vi "Climb Loop.vi"(0 "ClimbMotor":T12={"DeviceStatus"={"status"=FALSE, "code"=0, "source"=""}, "Type"=enum."PWM", "PWM"={"Digital Module"=enum."Digital Module 1", "PWM Channel"=enum."Invalid", "DeadBand"={"Name"="", "maxPositivePwm"=0, "minPositivePwm"=0, "centerPwm"=0, "maxNegativePwm"=0, "minNegativePwm"=0, "angularRange"=0}}, "CAN"={"Device Number"=0, "Control Mode"=enum."Percent VBus", "Semaphore"=refnum, "Max Vout"=12.0}, "Invert"=FALSE, "TransformRef"=refnum, "InvTransformRef"=refnum}, 1 "SkyHome":T7, 2 "Slapper":T9={"DevStatus"={"status"=FALSE, "code"=0, "source"=""}, "Solenoid Module"=enum."Solenoid Module 1", "Forward Solenoid Channel"=enum."Invalid", "Reverse Solenoid Channel"=enum."Invalid"}, 3 "Climb Step In":T1, 4 "Climb Step In2":T1, 5 "Time In":dbl, 6 "ClimbEncoder":T19={"DevStatus"={"status"=FALSE, "code"=0, "source"=""}, "EncoderIndex"=enum."Invalid", "CounterIndex"=enum."Invalid", "DistancePerCount"=1.0, "Decoding Type"=enum."4x"}, 7 "Rung counter in":i32, 8 "BrakeServo":T3={"DeviceStatus"={"status"=FALSE, "code"=0, "source"=""}, "Digital Module"=enum."Digital Module 1", "PWM Channel"=enum."Invalid", "DeadBand"={"Name"="", "maxPositivePwm"=0, "minPositivePwm"=0, "centerPwm"=0, "maxNegativePwm"=0, "minNegativePwm"=0, "angularRange"=0}}, 10 "PullUp":T9={"DevStatus"={"status"=FALSE, "code"=0, "source"=""}, "Solenoid Module"=enum."Solenoid Module 1", "Forward Solenoid Channel"=enum."Invalid", "Reverse Solenoid Channel"=enum."Invalid"}, 11 "array":i32[](array[numeric]), 12 "ClimbCurrent":T16, 13 "rt fifo":refnum<k33>, 15 "Auto Ascent Log Enable":bool=TRUE, 17 "time ref":dbl, 18 "Climb mode In":enum16{"Wait", "Automatic", "Manual", "Abort"}(ring)) -> (9 "Rung counter out":i32, 14 "Climb Step Out":T1, 16 "# elements":u32, 19 "Time Out":dbl)   [LabVIEW 2012]
uses:
  <vilib>/Rock Robotics/WPI/Encoder/WPI_EncoderDevRef.ctl
  <vilib>/Rock Robotics/SystemInterfaces/Encoder/FPGA_EncoderIdx.ctl
  <vilib>/Rock Robotics/SystemInterfaces/Counter/FPGA_CounterCtrSystemIndex.ctl
  <vilib>/Rock Robotics/WPI/Encoder/WPI_EncoderType.ctl
  <vilib>/Rock Robotics/WPI/AnalogChannel/WPI_AnalogChannelDevRef.ctl
  <vilib>/Rock Robotics/SystemInterfaces/Typedef/FPGA_TypedefAnalogModule.ctl
  <vilib>/Rock Robotics/SystemInterfaces/AI/FPGA_AIChannel.ctl
  <vilib>/Rock Robotics/WPI/Solenoid/WPI_SolenoidDevRef.ctl
  <vilib>/Rock Robotics/SystemInterfaces/Typedef/FPGA_TypedefSolenoidModule.ctl
  <vilib>/Rock Robotics/WPI/Solenoid/WPI_SolenoidChannel.ctl
  <vilib>/Rock Robotics/WPI/MotorControl/WPI_MotorControlDeviceRef.ctl
  <vilib>/Rock Robotics/SystemInterfaces/Typedef/FPGA_TypedefDigitalModule.ctl
  <vilib>/Rock Robotics/SystemInterfaces/DIO/FPGA_DIOPWMChannel.ctl
  <vilib>/Rock Robotics/WPI/PWM/WPI_PWMDeadband.ctl
  <vilib>/Rock Robotics/WPI/CAN/Jaguar/SubVIs/WPI_CANJaguar_ControlMode.ctl
  <vilib>/Rock Robotics/WPI/PWM/WPI_PWMTransform_ConPane.ctl
  climb_step_state.ctl
  <vilib>/Rock Robotics/WPI/DigitalInput/WPI_DigitalInputDevRef.ctl
  <vilib>/Rock Robotics/SystemInterfaces/DIO/FPGA_DIOChannel.ctl
  <vilib>/Rock Robotics/WPI/PWM/Servo/WPI_ServoDeviceRef.ctl
  <vilib>/Rock Robotics/WPI/Solenoid/WPI_SolenoidValue.ctl
  <vilib>/Rock Robotics/WPI/Solenoid/WPI_SolenoidSetEnum.vi
panel:
  out "Prev":T1
  in  "s":bool
  out "Current":dbl(graph)
  in  "Tab Control":T2(tab)
  in  "Auto Flip Speed":dbl=-0.2
  in  "distance to flip":dbl=-630.0
  in  "Man Flip Speed":dbl=-0.75
  out "Distance Flip":dbl
  in  "Target extend dist":dbl=1000.0
  in  "Motor Coerce":dbl=0.85
  out "At Lo":bool
  out "At Hi":bool
  in  "Near Limit":dbl=400.0
  in  "Speed near Lim Up":dbl=0.2
  in  "Precision":bool=TRUE
  out "Distance":dbl
  in  "Speed near Lim Dn":dbl=0.11
  out "state":bool
  in  "reset":bool
  in  "wait":dbl=2.0
  in  "Target extend dist 2":dbl=2735.0
  out "state 2":bool
  out "At Hi 2":bool
  out "At Lo 2":bool
  in  "Speed near Lim Dn 2":dbl=0.11
  out "Distance 2":dbl
  in  "Speed near Lim Up 2":dbl=0.2
  in  "Near Limit 2":dbl=400.0
  in  "Motor Coerce 2":dbl=0.85
  in  "Retract Test Dist":dbl=2450.0
  in  "delay post slap":dbl=2.0
  out "Auto Current":dbl(graph)
  in  "Current sensor load 2":dbl=0.5
  out "Voltage":dbl
  in  "Distance desired to\nretract tail hook completely 2":dbl=-650.0
  out "Distance Retracted":dbl
  out "Dist Used":dbl
  in  "L3 offset":dbl=20.0
  out "State":enum16{"Engaged", "Untension", "Disengaged"}(ring)
  in  "Brake Delay":dbl=0.2
  in  "Servo Disengage":i32
  in  "Untension Speed":dbl=-0.1
  in  "Reverse Time":dbl=0.4
  in  "Servo Engage":i32=120
  in  "Slow Retract":dbl=-0.25
  in  "Slow Extend":dbl=0.25
  in  "Climb Extend Speed":dbl=1.0
  in  "Climb Retract Speed":dbl=-0.9
  out "State 2":enum16{"Engaged", "Untension", "Disengaged"}(ring)
  in  "Servo Disengage 2":i32
  in  "Servo Engage 2":i32=120
  in  "Brake Delay 2":dbl=0.2
  in  "Reverse Time 2":dbl=0.4
  in  "Untension Speed 2":dbl=-0.1
  out "SkyHook is Home":bool
  out "Sky Enc":dbl
  out "Climb Started?":bool
  # "Encoder Displacement\n110 counts ~ 1 inch\n7 counts ~ 1/16 inch\n40 counts ~ Tooth-tooth on brake wheel"
  # "was -0.18 at Champs"
  # "It is a delay to allow the robot to stop \nswinging after a T-Rex pull-up, prior to \nextending the ShyHook to max distance.\n\nThis delay only affects level 2, not level 3."
  # "Distance desired to \nretract (enough to detect if\nwe have weight on current sensor\nin next case) 2"
  # "BRAKE"
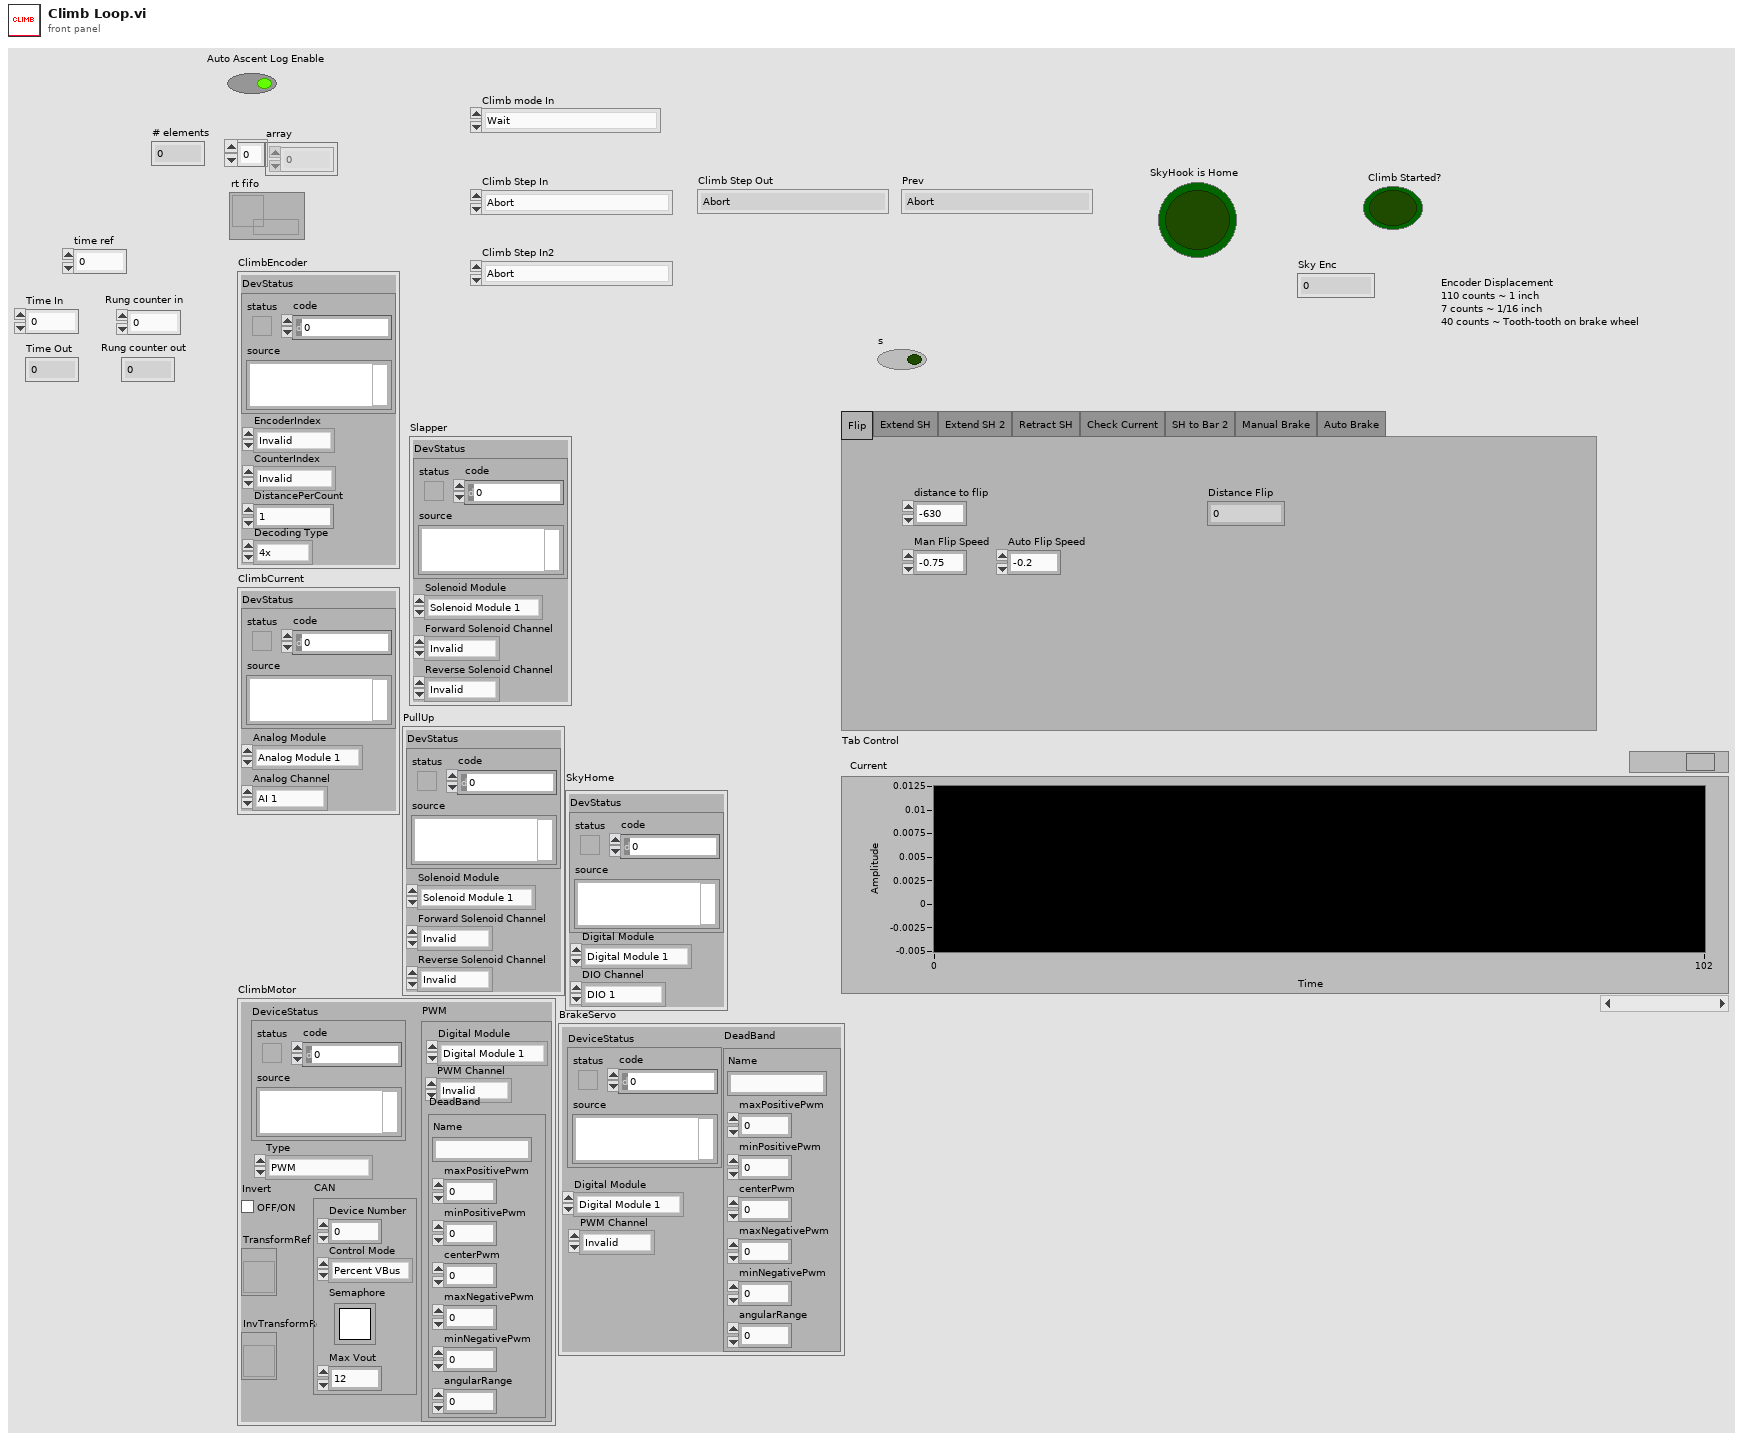
[diagram p1: front panel]
types:
  T1 = typedef "climb_step_state.ctl" = enum16{"Abort", "Approach Bar", "Approach +", "Climb Step 1", "Climb Step 2", "Climb Step 3", "Climb Step 4", "Climb Step 5", "Climb Step 6", "Climb Step 7", "Check Finished", "Check Continue"}
  T2 = enum32{"Flip", "Extend SH", "Extend SH 2", "Retract SH", "Check Current", "SH to Bar 2", "Manual Brake", "Auto Brake"}
  T3 = typedef "WPI_ServoDeviceRef.ctl" = cluster{"DeviceStatus":errorcluster, "Digital Module":T4, "PWM Channel":T5, "DeadBand":T6}
  T4 = typedef "FPGA_TypedefDigitalModule.ctl" = enum16{"Digital Module 1", "Digital Module 2"}
  T5 = typedef "FPGA_DIOPWMChannel.ctl" = enum8{"PWM 1", "PWM 2", "PWM 3", "PWM 4", "PWM 5", "PWM 6", "PWM 7", "PWM 8", "PWM 9", "PWM 10", "Invalid"}
  T6 = typedef "WPI_PWMDeadband.ctl" = cluster{"Name":string, "maxPositivePwm":i32, "minPositivePwm":i32, "centerPwm":i32, "maxNegativePwm":i32, "minNegativePwm":i32, "angularRange":u16}
  T7 = typedef "WPI_DigitalInputDevRef.ctl" = cluster{"DevStatus":errorcluster, "DIO Channel":T8, "Digital Module":T4}
  T8 = typedef "FPGA_DIOChannel.ctl" = enum8{"DIO 1", "DIO 2", "DIO 3", "DIO 4", "DIO 5", "DIO 6", "DIO 7", "DIO 8", "DIO 9", "DIO 10", "DIO 11", "DIO 12", "DIO 13", "DIO 14", "Invalid"}
  T9 = typedef "WPI_SolenoidDevRef.ctl" = cluster{"DevStatus":errorcluster, "Solenoid Module":T10, "Forward Solenoid Channel":T11, "Reverse Solenoid Channel":T11}
  T10 = typedef "FPGA_TypedefSolenoidModule.ctl" = enum16{"Solenoid Module 1", "Solenoid Module 2"}
  T11 = typedef "WPI_SolenoidChannel.ctl" = enum8{"Solenoid 1", "Solenoid 2", "Solenoid 3", "Solenoid 4", "Solenoid 5", "Solenoid 6", "Solenoid 7", "Solenoid 8", "Invalid"}
  T12 = typedef "WPI_MotorControlDeviceRef.ctl" = cluster{"DeviceStatus":errorcluster, "Type":enum16{"PWM", "CAN"}, "PWM":cluster{"Digital Module":T4, "PWM Channel":T5, "DeadBand":T6}, "CAN":cluster{"Device Number":u8, "Control Mode":T13, "Semaphore":T14, "Max Vout":dbl}, "Invert":bool, "TransformRef":T15, "InvTransformRef":T15}
  T13 = typedef "WPI_CANJaguar_ControlMode.ctl" = enum8{"Percent VBus", "Current", "Speed", "Position", "Voltage"}
  T14 = typedef "Semaphore RefNum" = refnum<k1>
  T15 = typedef "WPI_PWMTransform_ConPane.ctl" = refnum<vi>
  T16 = typedef "WPI_AnalogChannelDevRef.ctl" = cluster{"DevStatus":errorcluster, "Analog Module":T17, "Analog Channel":T18}
  T17 = typedef "FPGA_TypedefAnalogModule.ctl" = enum16{"Analog Module 1", "Analog Module 2"}
  T18 = typedef "FPGA_AIChannel.ctl" = enum8{"AI 1", "AI 2", "AI 3", "AI 4", "AI 5", "AI 6", "AI 7", "AI 8", "Invalid"}
  T19 = typedef "WPI_EncoderDevRef.ctl" = cluster{"DevStatus":errorcluster, "EncoderIndex":T20, "CounterIndex":T21, "DistancePerCount":dbl, "Decoding Type":T22}
  T20 = typedef "FPGA_EncoderIdx.ctl" = enum8{"Enc 0", "Enc 1", "Enc 2", "Enc 3", "Invalid"}
  T21 = typedef "FPGA_CounterCtrSystemIndex.ctl" = enum8{"Ctr 0", "Ctr 1", "Ctr 2", "Ctr 3", "Ctr 4", "Ctr 5", "Ctr 6", "Ctr 7", "Invalid"}
  T22 = typedef "WPI_EncoderType.ctl" = enum16{"1x", "2x", "4x"}
  T23 = typedef "WPI_SolenoidValue.ctl" = enum16{"Off", "On", "Forward", "Reverse"}
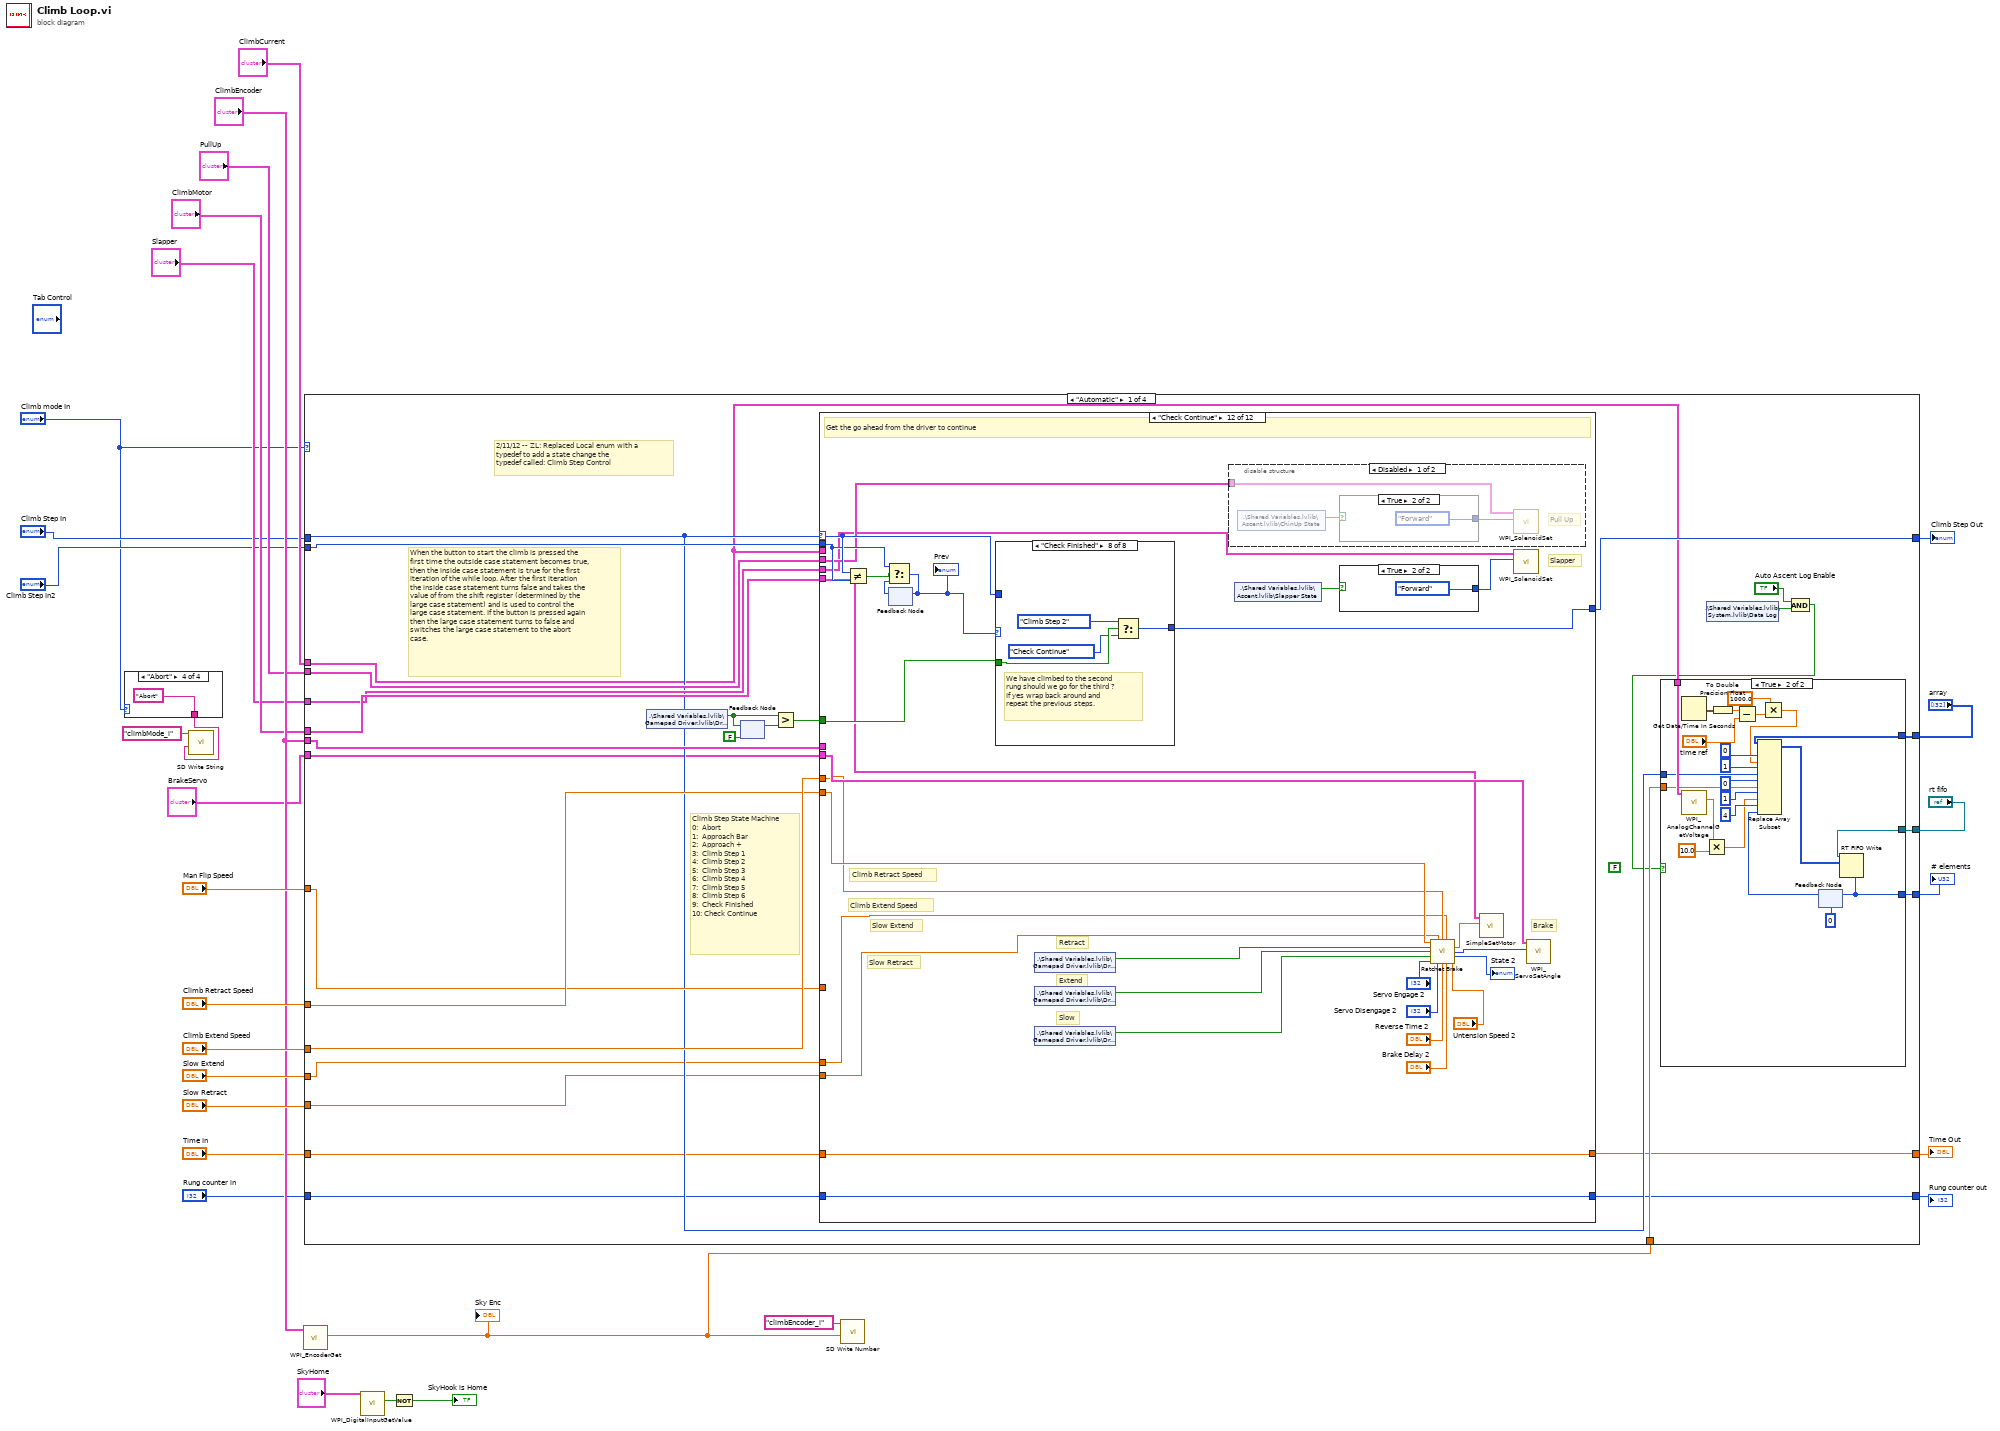
[diagram p0: block diagram]
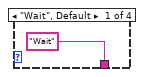
[diagram p2: hidden frame]
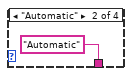
[diagram p3: hidden frame]
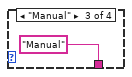
[diagram p4: hidden frame]
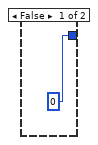
[diagram p5: hidden frame]
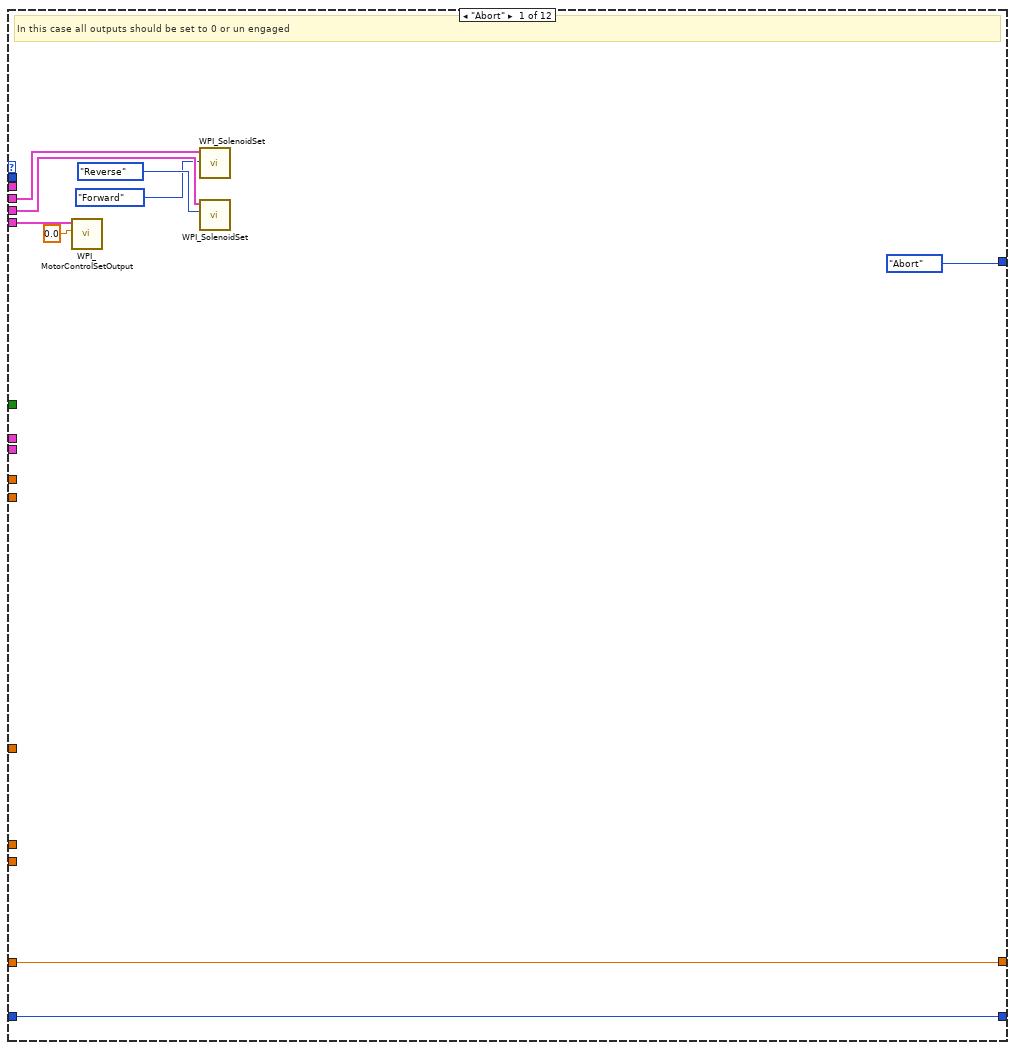
[diagram p6: hidden frame]
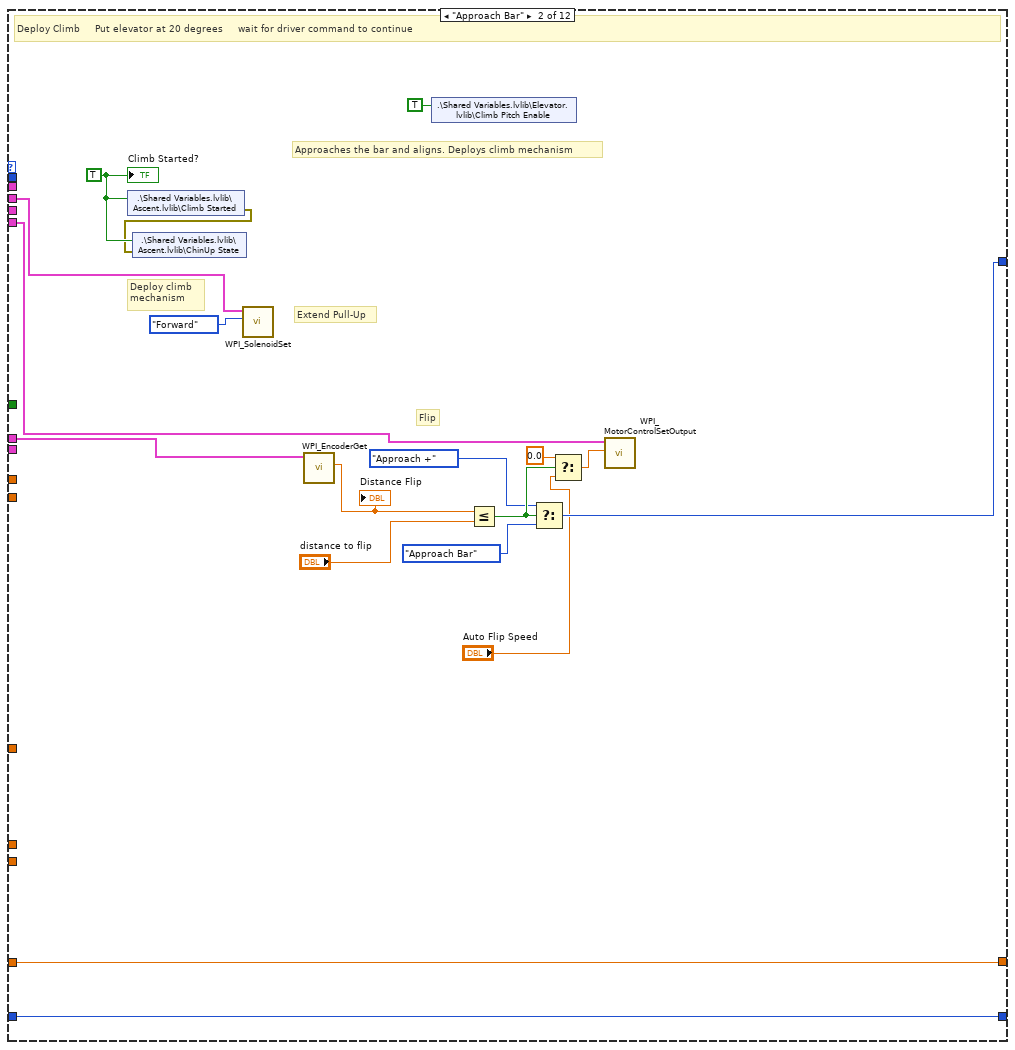
[diagram p7: hidden frame]
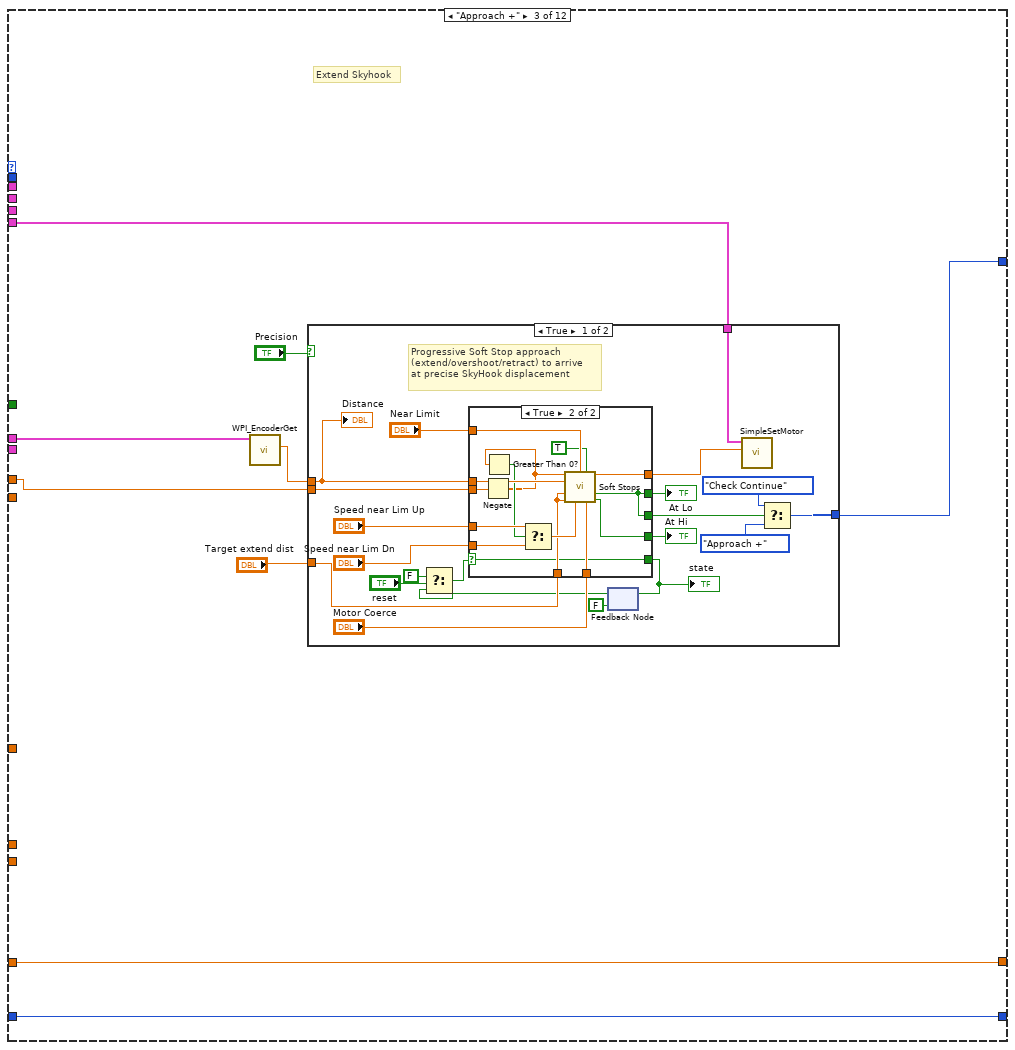
[diagram p8: hidden frame]
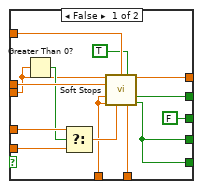
[diagram p9: hidden frame]
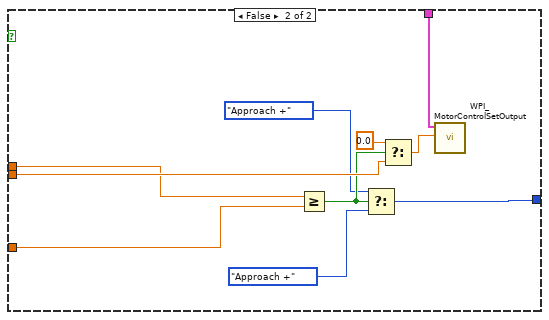
[diagram p10: hidden frame]
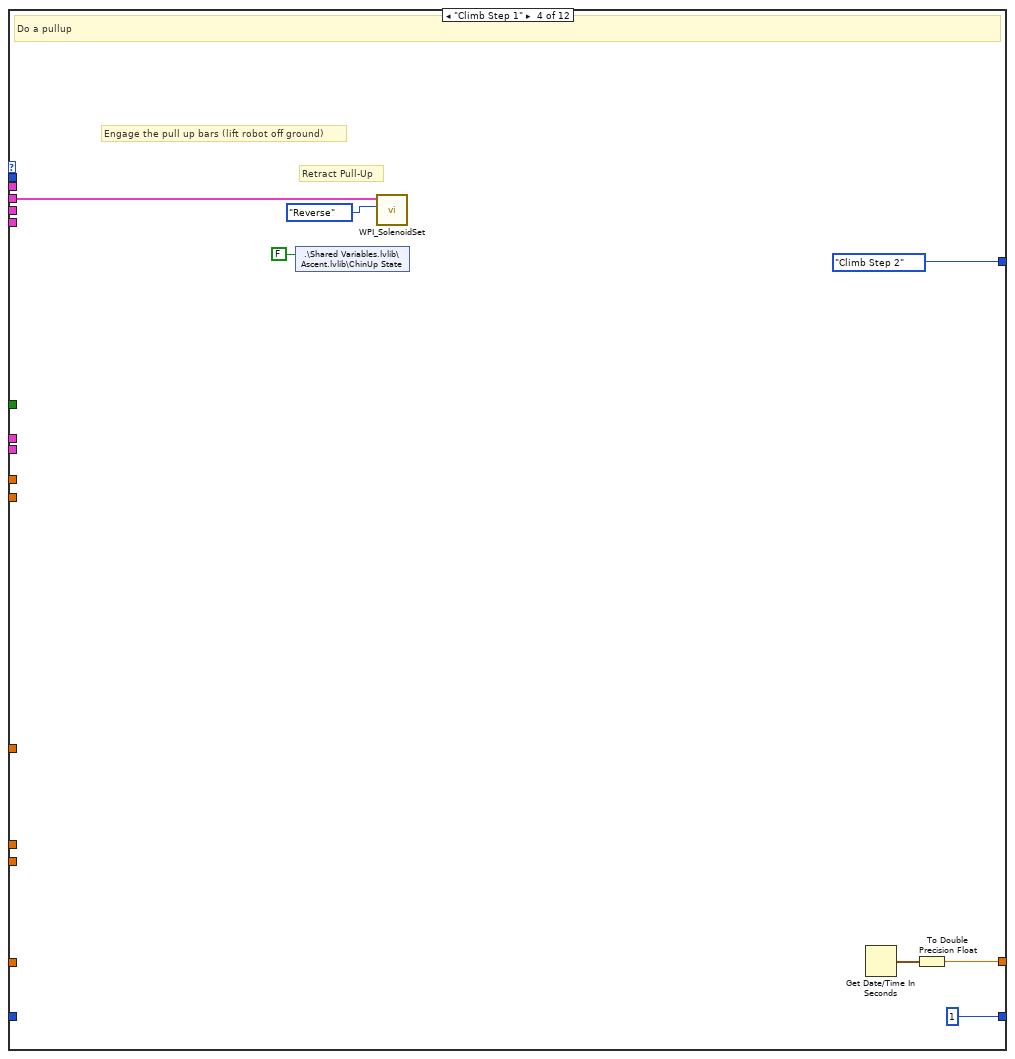
[diagram p11: hidden frame]
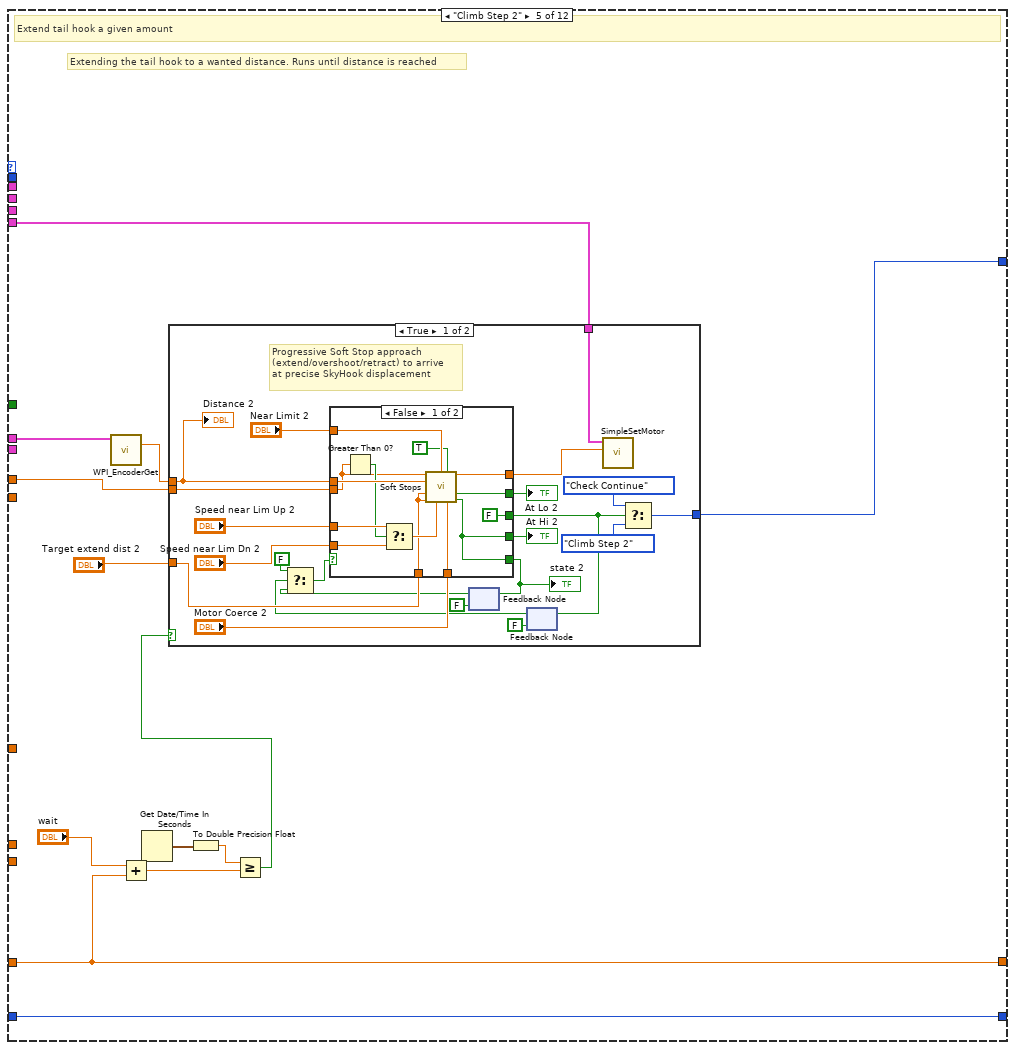
[diagram p12: hidden frame]
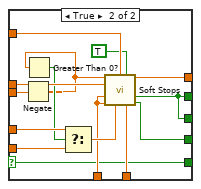
[diagram p13: hidden frame]
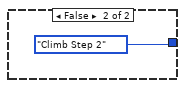
[diagram p14: hidden frame]
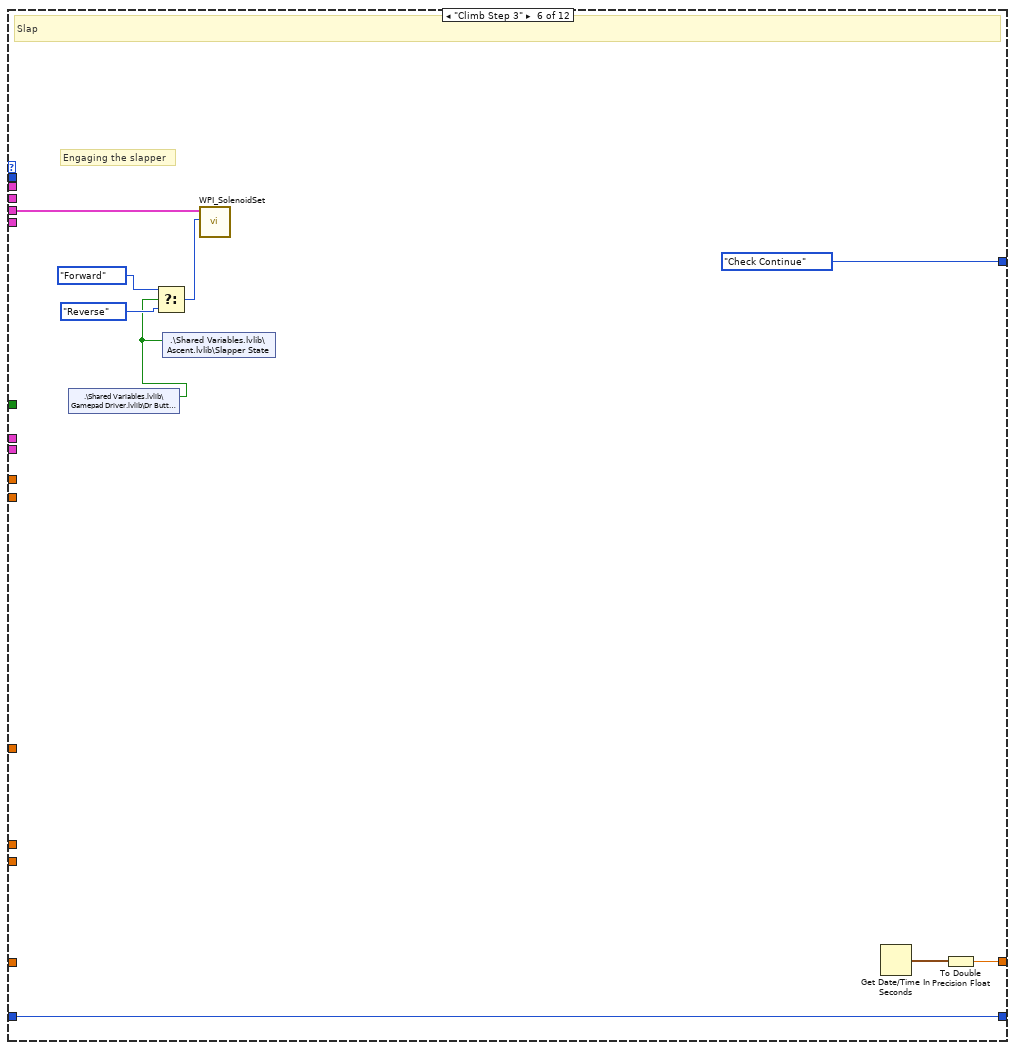
[diagram p15: hidden frame]
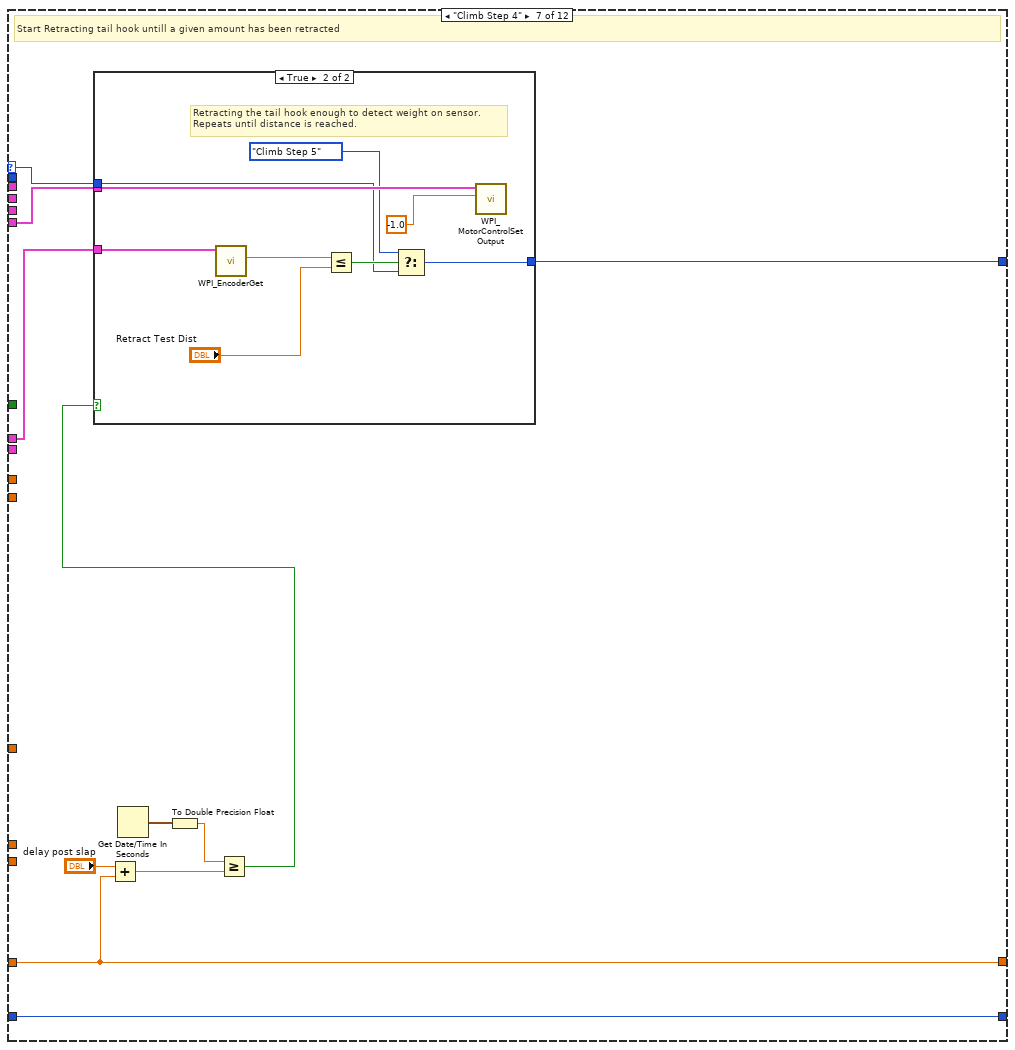
[diagram p16: hidden frame]
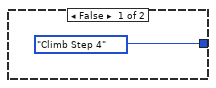
[diagram p17: hidden frame]
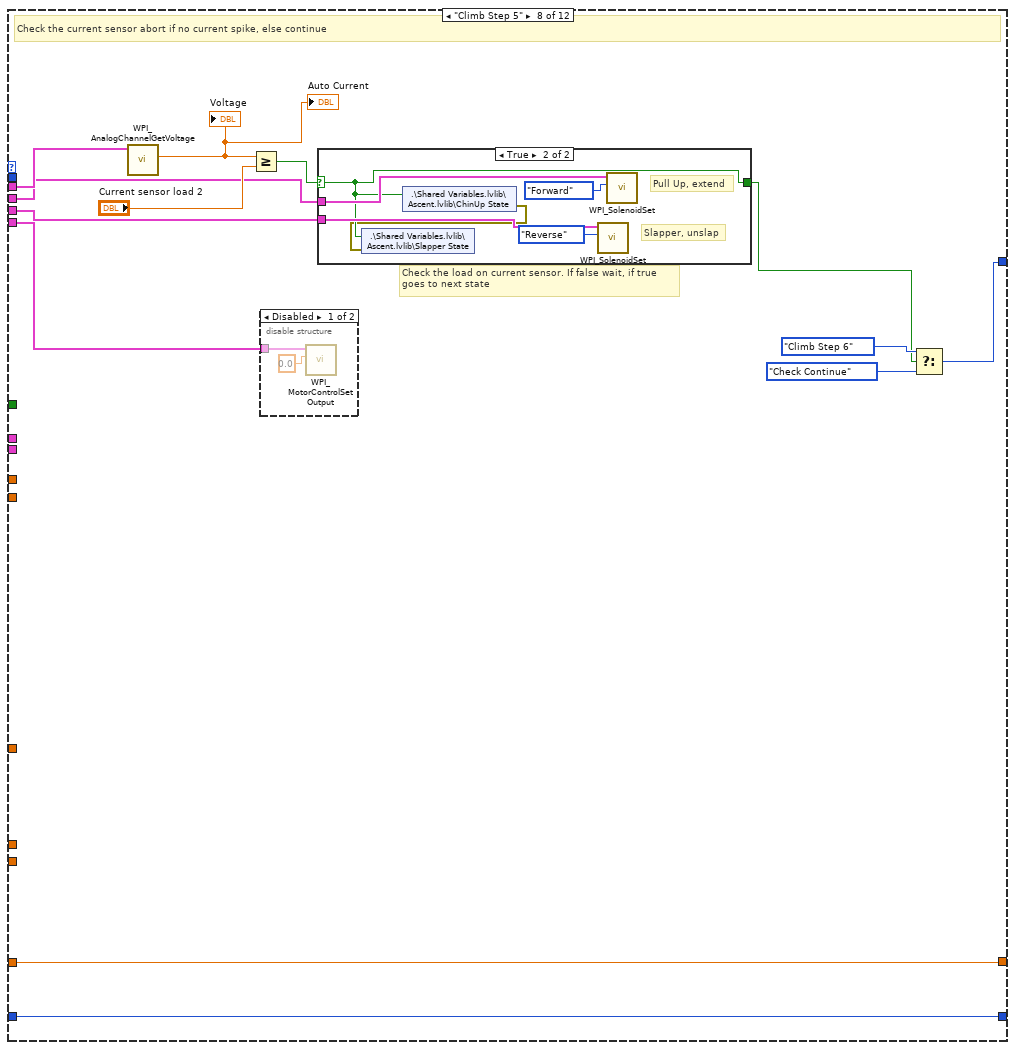
[diagram p18: hidden frame]
diagram:
  n1 = case shown="\"Abort\"" "Climb mode In" {
    tunnel: ["Wait" "Automatic" "Manual" "Abort"] -> w28
    frame "Wait", Default {
    }
    frame "Automatic" {
    }
    frame "Manual" {
    }
    frame "Abort" {
    }
  }
  n2 = call <vilib>:"SD Write String.vi"("String"=w28, "Name"="climbMode_i") -> ()  [unwired: 8 in, 2 out]
  n3 = call <vilib>:"WPI_EncoderGet.vi"("EncoderDevRef"="ClimbEncoder") -> ("Distance"=w1:dbl)  [unwired: 5 in, 5 out]
  "Sky Enc" <- w1
  n4 = case shown="\"Automatic\"" "Climb mode In" {
    tunnel: "PullUp" -> [w62 _ _ w438]
    tunnel: "ClimbMotor" -> [w61 _ _ w437]
    tunnel: "ClimbEncoder" -> [w60 _ _ _]
    tunnel: "Slapper" -> [w59 _ w421 w439]
    tunnel: "ClimbCurrent" -> [w43 _ _ w428]
    tunnel: [w58 climb_step_state."Abort" ("Climb Step") climb_step_state."Approach Bar" ("Climb Step") climb_step_state."Abort" ("Climb Step")] -> w13
    tunnel: "Climb Step In" -> [w45 _ _ _]
    tunnel: "Climb Step In2" -> [w57 _ _ _]
    tunnel: "Climb Extend Speed" -> [w56 _ _ w435]
    tunnel: "Climb Retract Speed" -> [w55 _ _ w434]
    tunnel: "Man Flip Speed" -> [w54 _ _ w433]
    tunnel: "Slow Extend" -> [w40 _ _ w432]
    tunnel: "Slow Retract" -> [w39 _ _ w431]
    tunnel: "BrakeServo" -> [w41 _ w420 w429]
    tunnel: "array" -> [w49 _ _ _]
    tunnel: [w48 u32 0 ("# elements") u32 0 ("# elements") u32 0 ("# elements")] -> w7
    tunnel: w1 -> [w44 _ _ _]
    tunnel: "rt fifo" -> [w42 _ _ _]
    tunnel: [w38 w413 w417 w425] -> w5
    tunnel: "Time In" -> [w37 w413 w417 w425]
    tunnel: [w36 w414 w418 w426] -> w3
    tunnel: "Rung counter in" -> [w35 w414 w418 w426]
    frame "Automatic" {
      (unwired) FALSE
      # "Climb Step State Machine\n0:  Abort\n1:  Approach Bar\n2:  Approach +\n3:  Climb Step 1\n4:  Climb Step 2\n5:  Climb Step 3\n6:  Climb Step 4\n7:  Climb Step 5\n8:  Climb Step 6\n9:  Check Finished\n10: Check Continue"
      # "2/11/12 -- ZL: Replaced Local enum with a \ntypedef to add a state change the \ntypedef called: Climb Step Control"
      # "When the button to start the climb is pressed the\nfirst time the outside case statement becomes true,\nthen the inside case statement is true for the first\niteration of the while loop. After the first iteration\nthe inside case statement turns false and takes the\nvalue of from the shift register (determined by the\nlarge case statement) and is used to control the \nlarge case statement. If the button is pressed again \nthen the large case statement turns to false and \nswitches the large case statement to the abort\ncase."
      n5 = shared-variable ".\\Shared Variables.lvlib\\Gamepad Driver.lvlib\\Dr Button 1"() -> (w53:bool)  [unwired: 1 in, 1 out]
      n6 = feedback-in #1(w53) -> ()
      n7 = feedback #1(FALSE ("Boolean")) -> (w52:bool)
      n8 = Greater?(x=w53, y=w52) -> (0:w51:bool)
      n9 = case shown="\"Check Continue\"" w45 {
        selector: w45 -> [_ _ _ _ _ _ w272 _ w319 _ _ w376]
        tunnel: w62 -> [w91 w113 _ w189 _ _ _ w293 w322 w336 _ w349]
        tunnel: [climb_step_state."Abort" ("Climb Step") w102 w116 climb_step_state."Climb Step 2" ("Climb Step") w190 climb_step_state."Check Continue" ("Climb Step") w273 w292 w320 w332 w342 w352] -> w58
        tunnel: w61 -> [w95 w111 w119 _ w193 _ w274 w286 w323 _ _ w357]
        tunnel: w60 -> [_ w110 w122 _ w192 _ w270 _ w326 _ _ _]
        tunnel: w59 -> [w93 _ _ _ _ w263 _ w294 _ _ _ w348]
        tunnel: w43 -> [_ _ _ _ _ _ _ w297 _ _ _ _]
        tunnel: w57 -> [_ _ _ _ _ _ _ _ _ _ _ w374]
        tunnel: w56 -> [_ _ w121 _ w191 _ _ _ _ _ _ w355]
        tunnel: w55 -> [_ _ _ _ _ _ _ _ _ _ _ w356]
        tunnel: w54 -> [_ _ _ _ _ _ _ _ _ _ _ _]
        tunnel: [w88 w99 w115 1 w202 w262 w271 w289 w315 w334 w340 w371] -> w36
        tunnel: w35 -> [w88 w99 w115 _ w202 w262 w271 w289 w315 w334 w341 w371]
        tunnel: [w87 w98 w114 w184 w197 w258 w269 w288 w318 w335 w339 w370] -> w38
        tunnel: w37 -> [w87 w98 w114 _ w197 _ w269 w288 w318 w335 w339 w370]
        tunnel: w51 -> [_ _ _ _ _ _ _ _ _ _ _ w369]
        tunnel: w41 -> [_ _ _ _ _ _ _ _ _ _ _ w358]
        tunnel: w40 -> [_ _ _ _ _ _ _ _ _ _ _ w354]
        tunnel: w39 -> [_ _ _ _ _ _ _ _ _ _ _ w353]
        frame "Abort" {
          # "In this case all outputs should be set to 0 or un engaged"
          n10 = call <vilib>:"WPI_MotorControlSetOutput.vi"("Output"=0.0, "MotorControlDevRef"=w95) -> ()  [unwired: 7 in, 3 out]
          n11 = call-poly <vilib>:"WPI_SolenoidSet.vi"("Value"=WPI_SolenoidValue."Forward", "SolenoidDevRef"=w91) -> ()  [unwired: 8 in, 2 out]
          n12 = call-poly <vilib>:"WPI_SolenoidSet.vi"("Value"=WPI_SolenoidValue."Reverse", "SolenoidDevRef"=w93) -> ()  [unwired: 8 in, 2 out]
        }
        frame "Approach Bar" {
          w97 = TRUE ("Climb Started?")
          # "Flip"
          # "Extend Pull-Up"
          # "Deploy climb \nmechanism"
          # "Approaches the bar and aligns. Deploys climb mechanism"
          # "Deploy Climb     Put elevator at 20 degrees     wait for driver command to continue"
          n13 = shared-variable ".\\Shared Variables.lvlib\\Ascent.lvlib\\Climb Started"(w97) -> (error out=w96:errorcluster)  [unwired: 1 in]
          n14 = shared-variable ".\\Shared Variables.lvlib\\Ascent.lvlib\\ChinUp State"(w97, error in=w96) -> ()  [unwired: 1 out]
          n15 = call-poly <vilib>:"WPI_SolenoidSet.vi"("Value"=WPI_SolenoidValue."Forward", "SolenoidDevRef"=w113) -> ()  [unwired: 8 in, 2 out]
          n16 = call <vilib>:"WPI_EncoderGet.vi"("EncoderDevRef"=w110) -> ("Distance"=w106:dbl)  [unwired: 5 in, 5 out]
          "Distance Flip" <- w106
          n17 = shared-variable ".\\Shared Variables.lvlib\\Elevator.lvlib\\Climb Pitch Enable"(TRUE ("Climb Pitch Enable")) -> ()  [unwired: 1 in, 1 out]
          n18 = Less Or Equal?(x=w106, y="distance to flip") -> (x <= y?=w105:bool)
          n19 = Select(t=climb_step_state."Approach +" ("Climb Step"), s=w105, f=climb_step_state."Approach Bar" ("Climb Step")) -> (s? t:f=w102:T1)
          n20 = Select(t=0.0, s=w105, f="Auto Flip Speed") -> (s? t:f=w107:dbl)
          n21 = call <vilib>:"WPI_MotorControlSetOutput.vi"("Output"=w107, "MotorControlDevRef"=w111) -> ()  [unwired: 7 in, 3 out]
          "Climb Started?" <- w97
        }
        frame "Approach +" {
          # "Extend Skyhook"
          n22 = call <vilib>:"WPI_EncoderGet.vi"("EncoderDevRef"=w122) -> ("Distance"=w120:dbl)  [unwired: 5 in, 5 out]
          n23 = case shown="True" "Precision" {
            tunnel: w121 -> [w131 w182]
            tunnel: w120 -> [w133 w181]
            tunnel: w119 -> [w140 w180]
            tunnel: "Target extend dist" -> [w132 w179]
            tunnel: [w141 w173] -> w116
            frame True {
              # "Progressive Soft Stop approach\n(extend/overshoot/retract) to arrive \nat precise SkyHook displacement"
              n24 = feedback #2(FALSE) -> (w124:bool)
              n25 = Select(t=FALSE, s="reset", f=w124) -> (s? t:f=w126:bool)
              n26 = case shown="True" w126 {
                selector: w126 -> [_ w162]
                tunnel: "Near Limit" -> [w157 w172]
                tunnel: "Motor Coerce" -> [w156 w171]
                tunnel: [FALSE ("At Hi") w160] -> w137
                tunnel: [w154 w169] -> w136
                tunnel: "Speed near Lim Up" -> [w152 w167]
                tunnel: "Speed near Lim Dn" -> [w151 w166]
                tunnel: w133 -> [w150 w165]
                tunnel: w132 -> [w148 w163]
                tunnel: w131 -> [w147 w159]
                tunnel: [w144 w162] -> w130
                tunnel: [w145 w160] -> w128
                tunnel: [w144 w161] -> w127
                frame False {
                  n27 = Greater Than 0?(x=w147) -> (x > 0?=w149:bool)
                  n28 = Select(t=w152, s=w149, f=w151) -> (s? t:f=w153:dbl)
                  n29 = call "Soft Stops.vi"("Motor In"=w147, "correlation"=TRUE, "Sense"=w150, "Lo Limit"=w148, "Hi Limit"=w148, "Speed near Limit"=w153, "Margin"=w157, "Motor Coerce"=w156) -> ("Motor Out"=w154:dbl, "At Lo"=w145:bool, "At Hi"=w144:bool)  [unwired: 5 in]
                }
                frame True {
                  n30 = Negate(x=w159) -> (-x=w158:dbl)
                  n31 = Greater Than 0?(x=w158) -> (x > 0?=w164:bool)
                  n32 = Select(t=w167, s=w164, f=w166) -> (s? t:f=w168:dbl)
                  n33 = call "Soft Stops.vi"("Motor In"=w158, "correlation"=TRUE, "Sense"=w165, "Lo Limit"=w163, "Hi Limit"=w163, "Speed near Limit"=w168, "Margin"=w172, "Motor Coerce"=w171) -> ("Motor Out"=w169:dbl, "At Lo"=w160:bool, "At Hi"=w161:bool)  [unwired: 5 in]
                }
              }
              "At Lo" <- w128
              "At Hi" <- w127
              "state" <- w130
              n34 = feedback-in #2(w130) -> ()
              n35 = call "SimpleSetMotor.vi"("Output"=w136, "MotorControlDevRef"=w140) -> ()  [unwired: 8 in, 2 out]
              n36 = Select(t=climb_step_state."Check Continue" ("Climb Step"), s=w137, f=climb_step_state."Approach +" ("Climb Step")) -> (s? t:f=w141:T1)
              "Distance" <- w133
            }
            frame False {
              n37 = Greater Or Equal?(x=w181, y=w179) -> (x >= y?=w176:bool)
              n38 = Select(t=climb_step_state."Approach +" ("Climb Step"), s=w176, f=climb_step_state."Approach +" ("Climb Step")) -> (s? t:f=w173:T1)
              n39 = Select(t=0.0, s=w176, f=w182) -> (s? t:f=w177:dbl)
              n40 = call <vilib>:"WPI_MotorControlSetOutput.vi"("Output"=w177, "MotorControlDevRef"=w180) -> ()  [unwired: 7 in, 3 out]
            }
          }
        }
        frame "Climb Step 1" {
          # "Retract Pull-Up"
          # "Engage the pull up bars (lift robot off ground)"
          # "Do a pullup"
          n41 = shared-variable ".\\Shared Variables.lvlib\\Ascent.lvlib\\ChinUp State"(FALSE ("ChinUp State")) -> ()  [unwired: 1 in, 1 out]
          n42 = call-poly <vilib>:"WPI_SolenoidSet.vi"("Value"=WPI_SolenoidValue."Reverse", "SolenoidDevRef"=w189) -> ()  [unwired: 8 in, 2 out]
          n43 = Get Date/Time In Seconds() -> (seconds since 1Jan1904=w185:timestamp)
          n44 = To Double Precision Float(number=w185) -> (double precision float=w184:dbl)
        }
        frame "Climb Step 2" {
          # "Extending the tail hook to a wanted distance. Runs until distance is reached"
          # "Extend tail hook a given amount"
          n45 = call <vilib>:"WPI_EncoderGet.vi"("EncoderDevRef"=w192) -> ("Distance"=w196:dbl)  [unwired: 5 in, 5 out]
          n46 = Add(x="wait", y=w197) -> (x+y=w199:dbl)
          n47 = Get Date/Time In Seconds() -> (seconds since 1Jan1904=w201:timestamp)
          n48 = To Double Precision Float(number=w201) -> (double precision float=w198:dbl)
          n49 = Greater Or Equal?(x=w198, y=w199) -> (x >= y?=w194:bool)
          n50 = case shown="True" w194 {
            tunnel: w191 -> [w213 _]
            tunnel: w196 -> [w215 _]
            tunnel: w193 -> [w221 _]
            tunnel: "Target extend dist 2" -> [w214 _]
            tunnel: [w222 climb_step_state."Climb Step 2" ("Climb Step")] -> w190
            frame True {
              # "Progressive Soft Stop approach\n(extend/overshoot/retract) to arrive \nat precise SkyHook displacement"
              n51 = feedback #3(FALSE) -> (w207:bool)
              n52 = feedback #4(FALSE) -> (w203:bool)
              n53 = Select(t=FALSE, s=w203, f=w207) -> (s? t:f=w208:bool)
              n54 = case shown="False" w208 {
                selector: w208 -> [_ w243]
                tunnel: "Near Limit 2" -> [w238 w253]
                tunnel: "Motor Coerce 2" -> [w237 w252]
                tunnel: [FALSE ("At Hi") w241] -> w204
                tunnel: [w235 w250] -> w218
                tunnel: "Speed near Lim Up 2" -> [w233 w248]
                tunnel: "Speed near Lim Dn 2" -> [w232 w247]
                tunnel: w215 -> [w231 w246]
                tunnel: w214 -> [w229 w244]
                tunnel: w213 -> [w228 w240]
                tunnel: [w225 w243] -> w212
                tunnel: [w226 w241] -> w210
                tunnel: [w225 w242] -> w209
                frame False {
                  n55 = Greater Than 0?(x=w228) -> (x > 0?=w230:bool)
                  n56 = Select(t=w233, s=w230, f=w232) -> (s? t:f=w234:dbl)
                  n57 = call "Soft Stops.vi"("Motor In"=w228, "correlation"=TRUE, "Sense"=w231, "Lo Limit"=w229, "Hi Limit"=w229, "Speed near Limit"=w234, "Margin"=w238, "Motor Coerce"=w237) -> ("Motor Out"=w235:dbl, "At Lo"=w226:bool, "At Hi"=w225:bool)  [unwired: 5 in]
                }
                frame True {
                  n58 = Negate(x=w240) -> (-x=w239:dbl)
                  n59 = Greater Than 0?(x=w239) -> (x > 0?=w245:bool)
                  n60 = Select(t=w248, s=w245, f=w247) -> (s? t:f=w249:dbl)
                  n61 = call "Soft Stops.vi"("Motor In"=w239, "correlation"=TRUE, "Sense"=w246, "Lo Limit"=w244, "Hi Limit"=w244, "Speed near Limit"=w249, "Margin"=w253, "Motor Coerce"=w252) -> ("Motor Out"=w250:dbl, "At Lo"=w241:bool, "At Hi"=w242:bool)  [unwired: 5 in]
                }
              }
              "At Lo 2" <- w210
              "At Hi 2" <- w209
              "state 2" <- w212
              n62 = feedback-in #3(w212) -> ()
              n63 = feedback-in #4(w204) -> ()
              n64 = call "SimpleSetMotor.vi"("Output"=w218, "MotorControlDevRef"=w221) -> ()  [unwired: 8 in, 2 out]
              n65 = Select(t=climb_step_state."Check Continue" ("Climb Step"), s=w204, f=climb_step_state."Climb Step 2" ("Climb Step")) -> (s? t:f=w222:T1)
              "Distance 2" <- w215
            }
            frame False {
            }
          }
        }
        frame "Climb Step 3" {
          # "Engaging the slapper"
          # "Slap"
          n66 = shared-variable ".\\Shared Variables.lvlib\\Gamepad Driver.lvlib\\Dr Button 12"() -> (w255:bool)  [unwired: 1 in, 1 out]
          n67 = Select(t=WPI_SolenoidValue."Forward" ("Value"), s=w255, f=WPI_SolenoidValue."Reverse" ("Value")) -> (s? t:f=w260:T23)
          n68 = shared-variable ".\\Shared Variables.lvlib\\Ascent.lvlib\\Slapper State"(w255) -> ()  [unwired: 1 in, 1 out]
          n69 = call-poly <vilib>:"WPI_SolenoidSet.vi"("Value"=w260, "SolenoidDevRef"=w263) -> ()  [unwired: 8 in, 2 out]
          n70 = Get Date/Time In Seconds() -> (seconds since 1Jan1904=w257:timestamp)
          n71 = To Double Precision Float(number=w257) -> (double precision float=w258:dbl)
        }
        frame "Climb Step 4" {
          # "Start Retracting tail hook untill a given amount has been retracted"
          n72 = Add(x="delay post slap", y=w269) -> (x+y=w267:dbl)
          n73 = Get Date/Time In Seconds() -> (seconds since 1Jan1904=w266:timestamp)
          n74 = To Double Precision Float(number=w266) -> (double precision float=w265:dbl)
          n75 = Greater Or Equal?(x=w265, y=w267) -> (x >= y?=w264:bool)
          n76 = case shown="True" w264 {
            tunnel: w274 -> [_ w284]
            tunnel: [climb_step_state."Climb Step 4" ("Climb Step") w281] -> w273
            tunnel: w272 -> [_ w279]
            tunnel: w270 -> [_ w276]
            frame False {
            }
            frame True {
              # "Retracting the tail hook enough to detect weight on sensor.\nRepeats until distance is reached."
              n77 = call <vilib>:"WPI_EncoderGet.vi"("EncoderDevRef"=w276) -> ("Distance"=w277:dbl)  [unwired: 5 in, 5 out]
              n78 = Less Or Equal?(x=w277, y="Retract Test Dist") -> (x <= y?=w282:bool)
              n79 = Select(t=climb_step_state."Climb Step 5" ("Climb Step"), s=w282, f=w279) -> (s? t:f=w281:T1)
              n80 = call <vilib>:"WPI_MotorControlSetOutput.vi"("Output"=-1.0 ("f"), "MotorControlDevRef"=w284) -> ()  [unwired: 7 in, 3 out]
            }
          }
        }
        frame "Climb Step 5" {
          # "Check the load on current sensor. If false wait, if true\ngoes to next state"
          # "Check the current sensor abort if no current spike, else continue"
          n81 = call <vilib>:"WPI_AnalogChannelGetVoltage.vi"("AIDeviceRef"=w297) -> ("Voltage"=w287:dbl)  [unwired: 8 in, 2 out]
          "Voltage" <- w287
          "Auto Current" <- w287
          n82 = Greater Or Equal?(x=w287, y="Current sensor load 2") -> (x >= y?=w295:bool)
          n83 = disable-structure shown="Disabled" {
            disable-tunnel: w286 -> [w298 _]
            frame Disabled {
              n84 = call <vilib>:"WPI_MotorControlSetOutput.vi"("Output"=0.0 ("f"), "MotorControlDevRef"=w298) -> ()  [unwired: 7 in, 3 out]
            }
            frame Enabled {
            }
          }
          n85 = case shown="True" w295 {
            selector: w295 -> [w300 w302]
            tunnel: w294 -> [_ w306]
            tunnel: w293 -> [_ w303]
            tunnel: [w300 w302] -> w290
            frame False {
            }
            frame True {
              # "Slapper, unslap"
              # "Pull Up, extend"
              n86 = shared-variable ".\\Shared Variables.lvlib\\Ascent.lvlib\\ChinUp State"(w302) -> (error out=w301:errorcluster)  [unwired: 1 in]
              n87 = shared-variable ".\\Shared Variables.lvlib\\Ascent.lvlib\\Slapper State"(w302, error in=w301) -> ()  [unwired: 1 out]
              n88 = call-poly <vilib>:"WPI_SolenoidSet.vi"("Value"=WPI_SolenoidValue."Reverse", "SolenoidDevRef"=w306) -> ()  [unwired: 8 in, 2 out]
              n89 = call-poly <vilib>:"WPI_SolenoidSet.vi"("Value"=WPI_SolenoidValue."Forward", "SolenoidDevRef"=w303) -> ()  [unwired: 8 in, 2 out]
            }
          }
          n90 = Select(t=climb_step_state."Climb Step 6" ("Climb Step"), s=w290, f=climb_step_state."Check Continue" ("Climb Step")) -> (s? t:f=w292:T1)
        }
        frame "Climb Step 6" {
          (unwired) climb_step_state."Check Finished" ("Climb Step")
          # "Temp Safety"
          # "Tail hook is retracted completely and pull up bar is engaged.\nWe are now hanging on rung 2 (if true). Repeats until true\nand then repeats process in order to climb to rung 3"
          # "Once fully retracted do another pullup"
          n91 = Equal?(x=1, y=w315) -> (x = y?=w310:bool)
          n92 = call <vilib>:"WPI_EncoderGet.vi"("EncoderDevRef"=w326) -> ("Distance"=w316:dbl)  [unwired: 5 in, 5 out]
          "Distance Retracted" <- w316
          n93 = Add(x="Distance desired to\nretract tail hook completely 2", y="L3 offset") -> (x+y=w308:dbl)
          n94 = Select(t="Distance desired to\nretract tail hook completely 2", s=w310, f=w308) -> (s? t:f=w311:dbl)
          "Dist Used" <- w311
          n95 = Less Or Equal?(x=w316, y=w311) -> (x <= y?=w312:bool)
          n96 = case shown="True" FALSE {
            selector: FALSE -> [w327 w330]
            tunnel: w322 -> [_ w331]
            tunnel: [w327 w330] -> _
            frame False {
            }
            frame True {
              # "Pull Up"
              n97 = shared-variable ".\\Shared Variables.lvlib\\Ascent.lvlib\\ChinUp State"(FALSE ("ChinUp State")) -> ()  [unwired: 1 in, 1 out]
              n98 = call-poly <vilib>:"WPI_SolenoidSet.vi"("Value"=WPI_SolenoidValue."Reverse", "SolenoidDevRef"=w331) -> ()  [unwired: 8 in, 2 out]
            }
          }
          n99 = Select(t=0.0, s=w312, f=-1.0) -> (s? t:f=w324:dbl)
          n100 = call <vilib>:"WPI_MotorControlSetOutput.vi"("Output"=w324, "MotorControlDevRef"=w323) -> ()  [unwired: 7 in, 3 out]
          n101 = Select(t=climb_step_state."Climb Step 7" ("Climb Step"), s=w312, f=w319) -> (s? t:f=w320:T1)
        }
        frame "Climb Step 7" {
          w332 = climb_step_state."Check Finished" ("Climb Step")
          # "Pull Up"
          n102 = call-poly <vilib>:"WPI_SolenoidSet.vi"("Value"=WPI_SolenoidValue."Reverse", "SolenoidDevRef"=w336) -> ()  [unwired: 8 in, 2 out]
          n103 = Select(t=w332, s="s", f=climb_step_state."Climb Step 7" ("Climb Step")) -> ()  [unwired: 1 out]
        }
        frame "Check Finished" {
          # "Rung counter keeps track of how many bars have been climbed.  Once rung counter reaches 3\nit aborts the climb because it has finished. If less than 3 it will go back to Step 2 to finish the climb"
          # "Check to see if we have climbed to level 3"
          n104 = Increment(x=w341) -> (x+1=w340:i32)
          n105 = Less?(x=w340, y=3) -> (x < y?=w345:bool)
          n106 = Select(t=climb_step_state."Check Continue" ("Climb Step"), s=w345, f=climb_step_state."Abort" ("Climb Step")) -> (s? t:f=w342:T1)
        }
        frame "Check Continue" {
          # "Slapper"
          # "Brake"
          # "Slow Retract"
          # "Slow Extend"
          # "Climb Extend Speed"
          # "Climb Retract Speed"
          # "Slow"
          # "Extend"
          # "Retract"
          # "Get the go ahead from the driver to continue"
          n107 = Not Equal?(x=w376, y=w374) -> (x != y?=w375:bool)
          n108 = feedback #5() -> (w372:T1)  [unwired: 1 in]
          n109 = Select(t=w374, s=w375, f=w372) -> (s? t:f=w373:T1)
          "Prev" <- w373
          n110 = feedback-in #5(w373) -> ()
          n111 = case shown="\"Check Finished\"" w373 {
            selector: w373 -> [w384 _ _ _ _ _ _ _]
            tunnel: w369 -> [_ w388 w392 w395 w397 w401 w405 w411]
            tunnel: [w384 w386 w389 w394 w398 w402 w406 w410] -> w352
            tunnel: w376 -> [_ w385 w391 _ _ _ _ _]
            frame "Abort", Default {
              # "This is a final case once here\n you are done in automatic mode"
            }
            frame "Approach Bar" {
              # "This Case not exercised in \nCheck Continue, since \nApproach + happens \nimmediately after \nApproach Bar"
              # "The climb mechinism is now folded \nout, and we are awaiting the driver \nto tell us that its ok to do the first \nchin up ie 10 point climb"
              n112 = Select(t=climb_step_state."Climb Step 1" ("Climb Step"), s=w388, f=w385) -> (s? t:f=w386:T1)
            }
            frame "Approach +" {
              n113 = Select(t=climb_step_state."Climb Step 1" ("Climb Step"), s=w392, f=w391) -> (s? t:f=w389:T1)
            }
            frame "Climb Step 1" {
              # "We are hanging off the first rung\nshould we attempt the second"
              n114 = Select(t=climb_step_state."Climb Step 2" ("Climb Step"), s=w395, f=climb_step_state."Check Continue" ("Climb Step")) -> (s? t:f=w394:T1)
            }
            frame "Climb Step 2" {
              # "Observe if extension correct for Slap,\nand/or synch with gyro swing."
              n115 = Select(t=climb_step_state."Climb Step 3" ("Climb Step"), s=w397, f=climb_step_state."Check Continue" ("Climb Step")) -> (s? t:f=w398:T1)
            }
            frame "Climb Step 3" {
              # "Decide if Slap looks good."
              n116 = Select(t=climb_step_state."Climb Step 4" ("Climb Step"), s=w401, f=climb_step_state."Check Continue" ("Climb Step")) -> (s? t:f=w402:T1)
            }
            frame "Climb Step 5" {
              # "Correct problem with \nno load on SkyHook.\nRe-position & re-slap."
              n117 = Select(t=climb_step_state."Climb Step 4" ("Climb Step"), s=w405, f=climb_step_state."Check Continue" ("Climb Step")) -> (s? t:f=w406:T1)
            }
            frame "Check Finished" {
              # "We have climbed to the second \nrung should we go for the third ?\nIf yes wrap back around and \nrepeat the previous steps."
              n118 = Select(t=climb_step_state."Climb Step 2" ("Climb Step"), s=w411, f=climb_step_state."Check Continue" ("Climb Step")) -> (s? t:f=w410:T1)
            }
          }
          n119 = shared-variable ".\\Shared Variables.lvlib\\Gamepad Driver.lvlib\\Dr Button 6"() -> (w367:bool)  [unwired: 1 in, 1 out]
          n120 = shared-variable ".\\Shared Variables.lvlib\\Gamepad Driver.lvlib\\Dr Button 5"() -> (w366:bool)  [unwired: 1 in, 1 out]
          n121 = shared-variable ".\\Shared Variables.lvlib\\Gamepad Driver.lvlib\\Dr Button 7"() -> (w365:bool)  [unwired: 1 in, 1 out]
          n122 = disable-structure shown="Disabled" {
            disable-tunnel: w349 -> [w377 _]
            frame Disabled {
              # "Pull Up"
              n123 = shared-variable ".\\Shared Variables.lvlib\\Ascent.lvlib\\ChinUp State"() -> (w378:bool)  [unwired: 1 in, 1 out]
              n124 = case shown="True" w378 {
                tunnel: [WPI_SolenoidValue."Reverse" ("Value") WPI_SolenoidValue."Forward" ("Value")] -> w379
                frame False {
                }
                frame True {
                }
              }
              n125 = call-poly <vilib>:"WPI_SolenoidSet.vi"("Value"=w379, "SolenoidDevRef"=w377) -> ()  [unwired: 8 in, 2 out]
            }
            frame Enabled {
            }
          }
          n126 = shared-variable ".\\Shared Variables.lvlib\\Ascent.lvlib\\Slapper State"() -> (w350:bool)  [unwired: 1 in, 1 out]
          n127 = case shown="True" w350 {
            tunnel: [WPI_SolenoidValue."Reverse" ("Value") WPI_SolenoidValue."Forward" ("Value")] -> w351
            frame False {
            }
            frame True {
            }
          }
          n128 = call "Ratchet Brake.vi"("Untension Speed"="Untension Speed 2", "Slow Extend"=w354, "Brake Delay"="Brake Delay 2", "Extend Speed"=w355, "Reverse Time"="Reverse Time 2", "Slow Retract"=w353, "Servo Disengage"="Servo Disengage 2", "Retract Speed"=w356, "Retract"=w367, "Extend"=w366, "Slow"=w365, "Servo Engage"="Servo Engage 2") -> ("Motor"=w359:dbl, "Brake Servo"=w347:i32, "State"=→"State 2":enum16{"Engaged", "Untension", "Disengaged"})  [unwired: 1 in]
          n129 = call "SimpleSetMotor.vi"("Output"=w359, "MotorControlDevRef"=w357) -> ()  [unwired: 8 in, 2 out]
          n130 = call-poly <vilib>:"WPI_SolenoidSet.vi"("Value"=w351, "SolenoidDevRef"=w348) -> ()  [unwired: 8 in, 2 out]
          n131 = call <vilib>:"WPI_ServoSetAngle.vi"("Angle"=w347, "ServoDeviceRef"=w358) -> ()  [unwired: 8 in, 2 out]
        }
      }
      n132 = shared-variable ".\\Shared Variables.lvlib\\System.lvlib\\Data Log"() -> (w46:bool)  [unwired: 1 in, 1 out]
      n133 = Compound Arithmetic op=AND("Auto Ascent Log Enable", w46) -> (w34:bool)
      n134 = case shown="True" w34 {
        tunnel: w49 -> [_ w80]
        tunnel: [u32 0 ("# elements") w79] -> w48
        tunnel: w45 -> [_ w74]
        tunnel: w44 -> [_ w75]
        tunnel: w43 -> [_ w78]
        tunnel: w42 -> [_ w70]
        frame False {
        }
        frame True {
          (unwired) 1 ("index")
          (unwired) 0 ("index")
          n135 = Get Date/Time In Seconds() -> (seconds since 1Jan1904=w73:timestamp)
          n136 = call <vilib>:"WPI_AnalogChannelGetVoltage.vi"("AIDeviceRef"=w78) -> ("Voltage"=w69:dbl)  [unwired: 8 in, 2 out]
          n137 = Multiply(x=w69, y=10.0) -> (x*y=w67:dbl)
          n138 = To Double Precision Float(number=w73) -> (double precision float=w72:dbl)
          n139 = Subtract(x=w72, y="time ref") -> (x-y=w66:dbl)
          n140 = Multiply(x=1000.0, y=w66) -> (x*y=w64:dbl)
          n141 = feedback #6(u32 0 ("# elements")) -> (w77:u32)
          n142 = Replace Array Subset(array=w80, new element #1=w64, index #1=0 ("index"), new element #2=w74, index #2=1 ("index"), new element #3=w75, index #3=2 ("index"), new element #4=w67, index #4=3 ("index"), new element #5=w77, index #5=4 ("index")) -> (w82:i32[])
          n143 = RT FIFO Write(0:w70, 1:w82) -> (7:w79:u32)  [unwired: 3 in, 3 out]
          n144 = feedback-in #6(w79) -> ()
        }
      }
    }
    frame "Abort" {
    }
    frame "Wait", Default {
      # "Initialize Slapper to relax and Brake to disengage"
      # "Brake"
      # "Slapper"
      n145 = call-poly <vilib>:"WPI_SolenoidSet.vi"("Value"=WPI_SolenoidValue."Forward", "SolenoidDevRef"=w421) -> ()  [unwired: 8 in, 2 out]
      n146 = call <vilib>:"WPI_ServoSetAngle.vi"("Angle"=0, "ServoDeviceRef"=w420) -> ()  [unwired: 8 in, 2 out]
    }
    frame "Manual" {
      # "Only can manually \nclimb after climb has\nbeen activated"
      n147 = shared-variable ".\\Shared Variables.lvlib\\Ascent.lvlib\\Climb Started"() -> (w430:bool)  [unwired: 1 in, 1 out]
      n148 = case shown="True" w430 {
        tunnel: w439 -> [_ w465]
        tunnel: w438 -> [_ w462]
        tunnel: w437 -> [_ w457]
        tunnel: w435 -> [_ w454]
        tunnel: w434 -> [_ w452]
        tunnel: w433 -> [_ _]
        tunnel: w432 -> [_ w455]
        tunnel: w431 -> [_ w453]
        tunnel: w429 -> [_ w458]
        tunnel: w428 -> [_ w442]
        frame False {
        }
        frame True {
          # "Brake"
          # "Slow Retract"
          # "Slow Extend"
          # "Climb Extend Speed"
          # "Climb Retract Speed"
          # "Man Flip Speed"
          # "Slow"
          # "Extend"
          # "Retract"
          # "Slapper"
          # "Pull Up"
          n149 = shared-variable ".\\Shared Variables.lvlib\\Ascent.lvlib\\Slapper State"() -> (w461:bool)  [unwired: 1 in, 1 out]
          n150 = shared-variable ".\\Shared Variables.lvlib\\Ascent.lvlib\\ChinUp State"() -> (w460:bool)  [unwired: 1 in, 1 out]
          n151 = call <vilib>:"WPI_AnalogChannelGetVoltage.vi"("AIDeviceRef"=w442) -> ("Voltage"=→"Current":dbl)  [unwired: 8 in, 2 out]
          n152 = shared-variable ".\\Shared Variables.lvlib\\Gamepad Driver.lvlib\\Dr Button 6"() -> (w451:bool)  [unwired: 1 in, 1 out]
          n153 = shared-variable ".\\Shared Variables.lvlib\\Gamepad Driver.lvlib\\Dr Button 5"() -> (w450:bool)  [unwired: 1 in, 1 out]
          n154 = shared-variable ".\\Shared Variables.lvlib\\Gamepad Driver.lvlib\\Dr Button 7"() -> (w449:bool)  [unwired: 1 in, 1 out]
          n155 = case shown="False" w460 {
            tunnel: [WPI_SolenoidValue."Reverse" ("Value") WPI_SolenoidValue."Forward" ("Value")] -> w463
            frame False {
            }
            frame True {
            }
          }
          n156 = case shown="False" w461 {
            tunnel: [WPI_SolenoidValue."Reverse" ("Value") WPI_SolenoidValue."Forward" ("Value")] -> w464
            frame False {
            }
            frame True {
            }
          }
          n157 = call-poly <vilib>:"WPI_SolenoidSet.vi"("Value"=w463, "SolenoidDevRef"=w462) -> ()  [unwired: 8 in, 2 out]
          n158 = call-poly <vilib>:"WPI_SolenoidSet.vi"("Value"=w464, "SolenoidDevRef"=w465) -> ()  [unwired: 8 in, 2 out]
          n159 = shared-variable ".\\Shared Variables.lvlib\\Elevator.lvlib\\Climb Pitch Enable"(FALSE ("Climb Pitch Enable")) -> ()  [unwired: 1 in, 1 out]
          n160 = call "Ratchet Brake.vi"("Untension Speed"="Untension Speed", "Slow Extend"=w455, "Brake Delay"="Brake Delay", "Extend Speed"=w454, "Reverse Time"="Reverse Time", "Slow Retract"=w453, "Servo Disengage"="Servo Disengage", "Retract Speed"=w452, "Retract"=w451, "Extend"=w450, "Slow"=w449, "Servo Engage"="Servo Engage") -> ("Motor"=w443:dbl, "Brake Servo"=w440:i32, "State"=→"State":enum16{"Engaged", "Untension", "Disengaged"})  [unwired: 1 in]
          n161 = call "SimpleSetMotor.vi"("Output"=w443, "MotorControlDevRef"=w457) -> ()  [unwired: 8 in, 2 out]
          n162 = call <vilib>:"WPI_ServoSetAngle.vi"("Angle"=w440, "ServoDeviceRef"=w458) -> ()  [unwired: 8 in, 2 out]
        }
      }
    }
  }
  "Climb Step Out" <- w13
  "# elements" <- w7
  "Time Out" <- w5
  "Rung counter out" <- w3
  n163 = call <vilib>:"WPI_DigitalInputGetValue.vi"("DigitalInputDevRef"="SkyHome") -> ("Value"=w10:bool)  [unwired: 8 in, 2 out]
  n164 = Not(x=w10) -> (.not. x?=→"SkyHook is Home":bool)
  n165 = call <vilib>:"SD Write Number.vi"("Numeric"=w1, "Name"="climbEncoder_i") -> ()  [unwired: 8 in, 2 out]
